vi "ReferencesFGV.vi"(7 "Get/Set":enum16{"Get", "Set"}(ring), 8 "error in (no error)":errorcluster, 11 "VeriStand dotNET Refs":T1) -> (0 "error out":errorcluster, 3 "VeriStand dotNET Refs out":T1)   [LabVIEW 2015, in "ni-veristand-steps-runtime-lib.lvlib"]
uses:
  ni-veristand-steps-runtime-lib.lvlib
  controls/VeriStand dotNet References.ctl
  NationalInstruments.VeriStand.ClientAPI
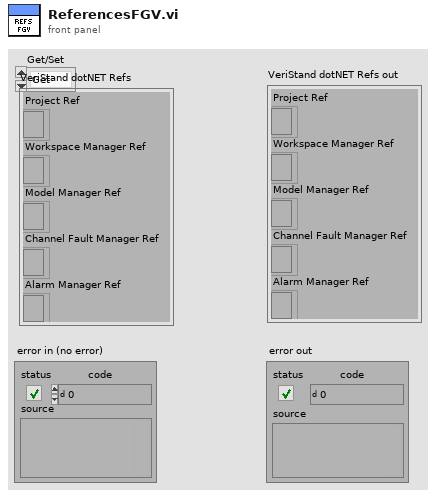
[diagram p1: front panel]
types:
  T1 = typedef "ni-veristand-steps-runtime-lib.lvlib/VeriStand dotNet References.ctl" = cluster{"Project Ref":refnum<k24>, "Workspace Manager Ref":refnum<k24>, "Model Manager Ref":refnum<k24>, "Channel Fault Manager Ref":refnum<k24>, "Alarm Manager Ref":refnum<k24>}
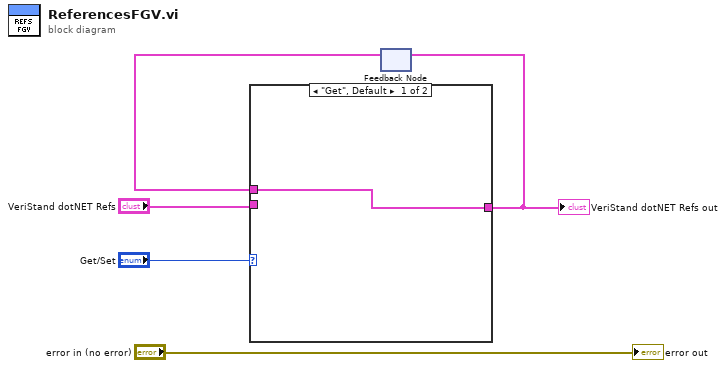
[diagram p0: block diagram]
diagram:
  n1 = feedback #1() -> (w4:T1)  [unwired: 1 in]
  n2 = case shown="\"Get\", Default" "Get/Set" {
    tunnel: "VeriStand dotNET Refs" -> [_ w7]
    tunnel: [w6 w7] -> w1
    tunnel: w4 -> [w6 _]
    frame "Get", Default {
    }
    frame "Set" {
    }
  }
  "VeriStand dotNET Refs out" <- w1
  n3 = feedback-in #1(w1) -> ()
  "error out" <- "error in (no error)"
